vi "Add Device to Stack.vi"(7 "Device in":refnum<class "Device.lvclass">, 8 "error in (no error)":errorcluster, 9 "Device UID":string, 11 "IP Connection in":refnum<class "IP Connection.lvclass">) -> (0 "error out":errorcluster, 3 "Device out":refnum<class "Device.lvclass">)   [LabVIEW 2011, in "Tinkerforge.lvlib" / "Device.lvclass"]
doc: "This VI adds the device to the stack after all preconditions are checked."
uses:
  Device.lvclass
  IP Connection/IP Connection.lvclass
  IP Connection/Type Definitions/Errors.ctl
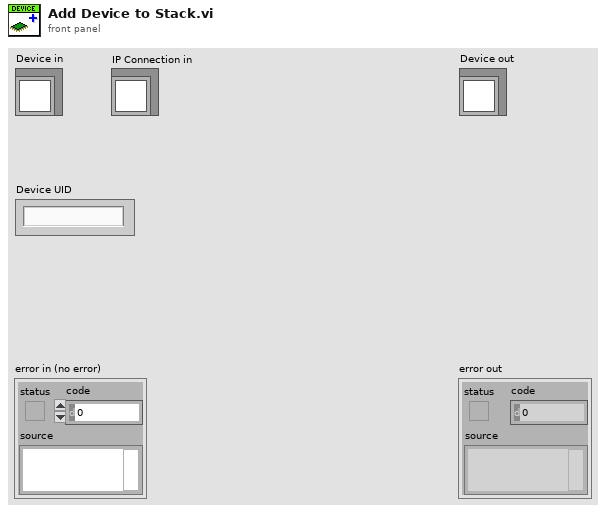
[diagram p1: front panel]
types:
  T1 = typedef "Tinkerforge.lvlib/IP Connection.lvclass/Errors.ctl" = enum16{"Timeout", "Device type incorrect", "Device already added", "Device not existing"}
  T2 = typedef "Tinkerforge.lvlib/IP Connection.lvclass/Get Stack ID Response.ctl" = cluster{"UID":string, "Firmware Version":T3, "Name":string, "Stack ID":u8}
  T3 = typedef "Tinkerforge.lvlib/Device.lvclass/Firmware Version.ctl" = cluster{"Major":u8, "Minor":u8, "Fix":u8}
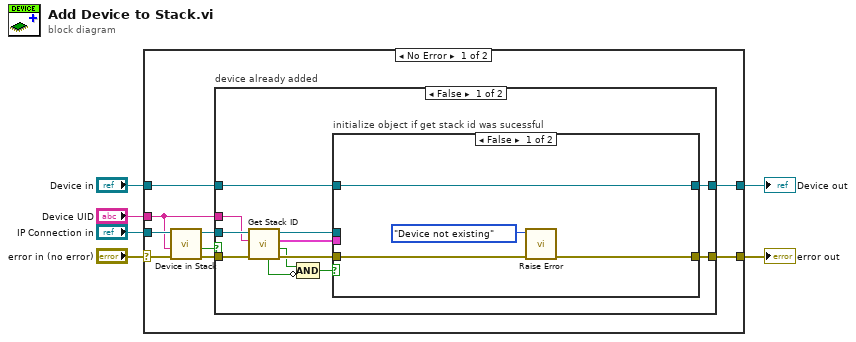
[diagram p0: block diagram]
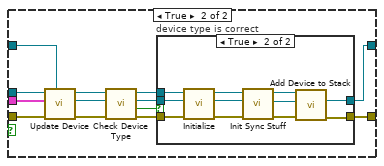
[diagram p2: hidden frame]
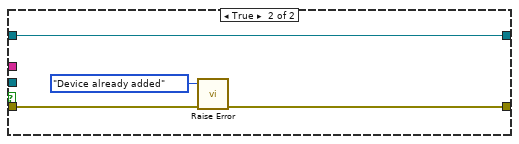
[diagram p4: hidden frame]
diagram:
  n1 = case shown="No Error" "error in (no error)" {
    selector: "error in (no error)" -> [w12 w60]
    tunnel: [w7 w60] -> w5
    tunnel: [w8 w59] -> w3
    tunnel: "Device in" -> [w9 w59]
    tunnel: "IP Connection in" -> [w11 _]
    tunnel: "Device UID" -> [w10 _]
    frame No Error {
      n2 = call "Device in Stack.vi"("error in (no error)"=w12, "Device UID"=w10, "IP Connection in"=w11) -> ("error out"=w14:errorcluster, "Device already in Stack"=w15:bool, "IP Connection out"=w13:refnum<class "IP Connection.lvclass">)  [unwired: 6 in]
      n3 = case "device already added" shown="False" w15 {
        tunnel: w14 -> [w27 w57]
        tunnel: w13 -> [w26 _]
        tunnel: w10 -> [w25 _]
        tunnel: w9 -> [w19 w58]
        tunnel: [w17 w56] -> w7
        tunnel: [w16 w58] -> w8
        frame False {
          n4 = call "Get Stack ID.vi"("error in (no error)"=w27, "Device UID"=w25, "IP Connection in"=w26) -> ("error out"=w24:errorcluster, "Sucessful"=w23:bool, "Get Stack ID Response"=w20:T2, "IP Connection out"=w18:refnum<class "IP Connection.lvclass">, "timed out"=w22:bool)  [unwired: 4 in]
          n5 = Compound Arithmetic op=AND(w23, invert w22) -> (w21:bool)
          n6 = case "initialize object if get stack id was sucessful" shown="False" w21 {
            tunnel: w24 -> [w30 w42]
            tunnel: w20 -> [_ w41]
            tunnel: w19 -> [w31 w40]
            tunnel: w18 -> [_ w39]
            tunnel: [w29 w38] -> w17
            tunnel: [w31 w37] -> w16
            frame False {
              n7 = call "Raise Error.vi"("Error In"=w30, "Error"=Errors."Device not existing") -> ("Error Out"=w29:errorcluster)  [unwired: 9 in]
            }
            frame True {
              n8 = call "Update Device.vi"("Device in"=w40, "error in (no error)"=w42, "Get Stack ID Response"=w41) -> ("error out"=w36:errorcluster, "Device out"=w34:refnum<class "Device.lvclass">)  [unwired: 7 in]
              n9 = call-dynamic "Check Device Type.vi"("error in (no error)"=w36, "Device in"=w34) -> ("error out"=w35:errorcluster, "correct Device"=w32:bool, "Device out"=w33:refnum<class "Device.lvclass">)  [unwired: 7 in]
              n10 = case "device type is correct" shown="True" w32 {
                tunnel: w39 -> [_ w54]
                tunnel: [w44 w51] -> w38
                tunnel: [w43 w50] -> w37
                tunnel: w35 -> [w44 w53]
                tunnel: w33 -> [w43 w52]
                frame False {
                }
                frame True {
                  n11 = call "Initialize.vi"("error in (no error)"=w53, "Device in"=w52, "IP Connection in"=w54) -> ("error out"=w49:errorcluster, "Device out"=w46:refnum<class "Device.lvclass">, "IP Connection out"=w45:refnum<class "IP Connection.lvclass">)  [unwired: 6 in]
                  n12 = call-dynamic "Init Sync Stuff.vi"("error in (no error)"=w49, "Device in"=w46) -> ("error out"=w48:errorcluster, "Device out"=w47:refnum<class "Device.lvclass">)  [unwired: 8 in]
                  n13 = call "Add Device to Stack.vi"("error in (no error)"=w48, "Device in"=w47, "IP Connection in"=w45) -> ("error out"=w51:errorcluster, "Device out"=w50:refnum<class "Device.lvclass">)  [unwired: 6 in, 1 out]
                }
              }
            }
          }
        }
        frame True {
          n14 = call "Raise Error.vi"("Error In"=w57, "Error"=Errors."Device already added") -> ("Error Out"=w56:errorcluster)  [unwired: 9 in]
        }
      }
    }
    frame Error {
    }
  }
  "error out" <- w5
  "Device out" <- w3
